vi "3 motor nonloop.vi"(8 "Error In":errorcluster, 9 "Reset":bool, 10 "speed":dbl[](array[numeric]), 11 "Array":refnum<class "Motor single.lvclass">[](array[class])) -> (0 "error out":errorcluster, 1 "encoder":i32[](array[numeric]), 2 "setpoint":dbl[](array[numeric]), 3 "appended array":refnum<class "Motor single.lvclass">[](array[class]), 4 "PID out":dbl[](array[numeric]))   [LabVIEW 2019]
uses:
  motor single class/Motor single.lvclass
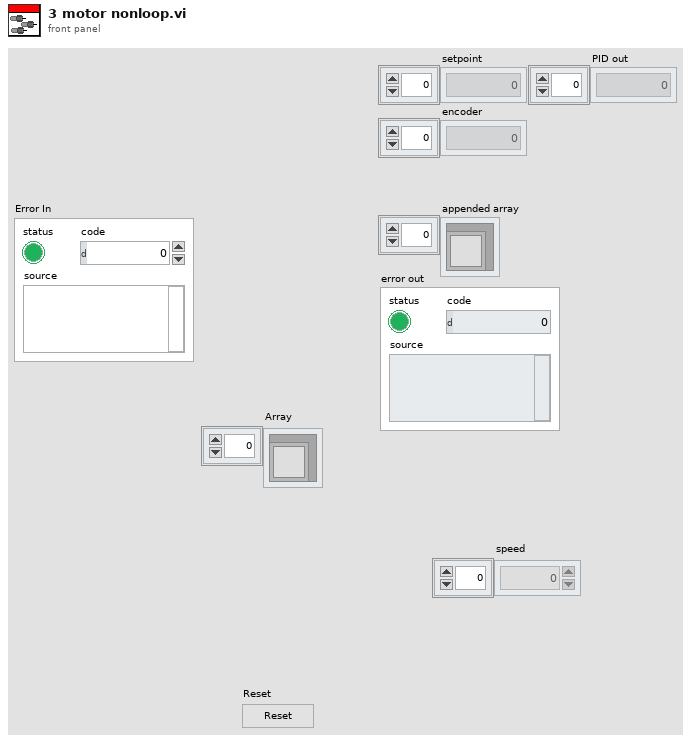
[diagram p1: front panel]
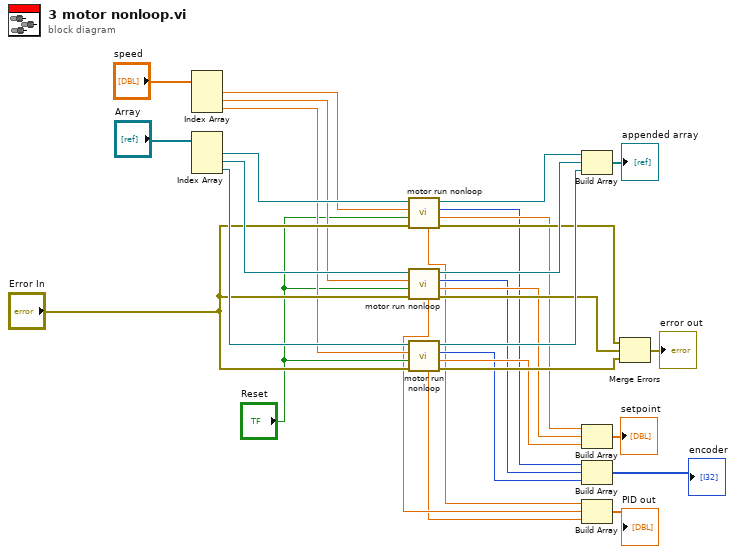
[diagram p0: block diagram]
diagram:
  n1 = Index Array(array="speed") -> (element #1=w24:dbl, element #2=w23:dbl, element #3=w22:dbl)  [unwired: 3 in]
  n2 = Index Array(array="Array") -> (element #1=w27:refnum<class "Motor single.lvclass">, element #2=w28:refnum<class "Motor single.lvclass">, element #3=w29:refnum<class "Motor single.lvclass">)  [unwired: 3 in]
  n3 = call "motor run nonloop.vi"("Error In"="Error In", "Reset"="Reset", "Speed (RPM)"=w24, "Motor single.lvclass"=w27) -> ("error out"=w16:errorcluster, "setpoint"=w12:dbl, "encoder out"=w9:i32, "output cluster"=w18:refnum<class "Motor single.lvclass">, "PID output"=w6:dbl)  [unwired: 3 in]
  n4 = call "motor run nonloop.vi"("Error In"="Error In", "Reset"="Reset", "Speed (RPM)"=w23, "Motor single.lvclass"=w28) -> ("error out"=w15:errorcluster, "setpoint"=w11:dbl, "encoder out"=w8:i32, "output cluster"=w19:refnum<class "Motor single.lvclass">, "PID output"=w5:dbl)  [unwired: 3 in]
  n5 = call "motor run nonloop.vi"("Error In"="Error In", "Reset"="Reset", "Speed (RPM)"=w22, "Motor single.lvclass"=w29) -> ("error out"=w14:errorcluster, "setpoint"=w10:dbl, "encoder out"=w7:i32, "output cluster"=w20:refnum<class "Motor single.lvclass">, "PID output"=w4:dbl)  [unwired: 3 in]
  n6 = Build Array(w18, w19, w20) -> (→"appended array":refnum<class "Motor single.lvclass">[])
  n7 = Build Array(w12, w11, w10) -> (→"setpoint":dbl[])
  n8 = Build Array(w9, w8, w7) -> (→"encoder":i32[])
  n9 = Build Array(w6, w5, w4) -> (→"PID out":dbl[])
  n10 = Merge Errors(w16, w15, w14) -> (→"error out":errorcluster)
